vi "ApproveZCoord (SubVI).vi"(8 "Zhigh":dbl, 9 "Zlow":dbl, 11 "Go to Z":dbl) -> (3 "Pass Z?":bool)   [LabVIEW 2016]
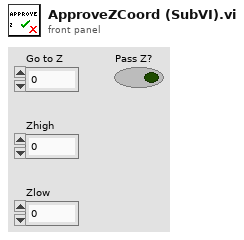
[diagram p1: front panel]
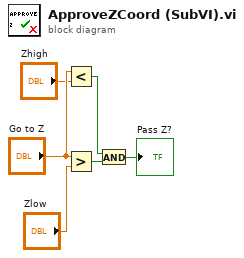
[diagram p0: block diagram]
diagram:
  n1 = Less?(x="Go to Z", y="Zhigh") -> (x < y?=w3:bool)
  n2 = Greater?(x="Go to Z", y="Zlow") -> (0:w2:bool)
  n3 = And(x=w3, y=w2) -> (x .and. y?=→"Pass Z?":bool)
